vi "LV2 DVR Reference.vi"(0 "DVR Input":refnum<data-value>, 11 "Error in":errorcluster, 13 "Operation":T1) -> (4 "DVR Output":refnum<data-value>, 15 "Error out":errorcluster)   [LabVIEW 2020, in "DVR Access.lvlib"]
uses:
  DVR Access.lvlib
  Typedefs/LV2 Operations.ctl
  Typedefs/Data Cluster.ctl
  DVR Handson.lvlib
panel:
  # "LV2 DVR REFRENCE"
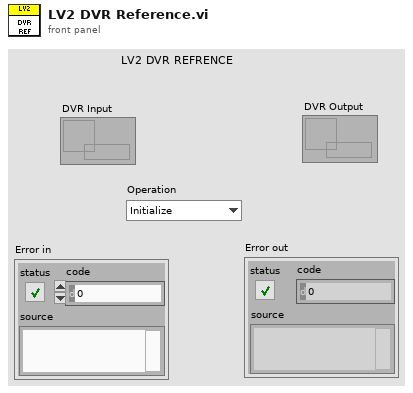
[diagram p1: front panel]
types:
  T1 = typedef "DVR Handson.lvlib/LV2 Operations.ctl" = enum16{"Initialize", "Read", "Write"}
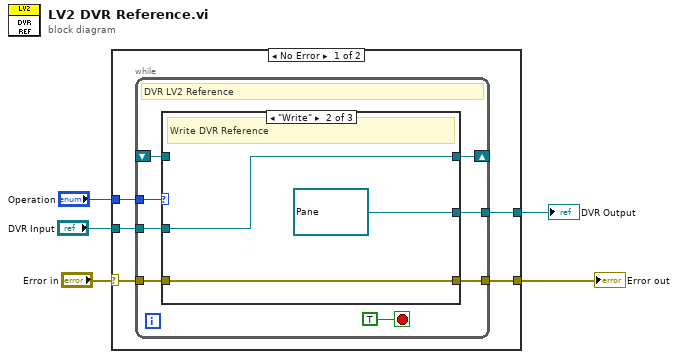
[diagram p0: block diagram]
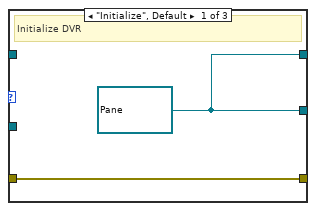
[diagram p2: hidden frame]
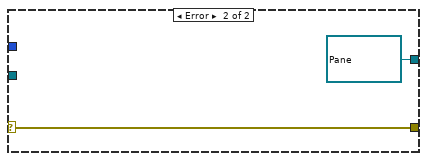
[diagram p4: hidden frame]
diagram:
  n1 = case shown="No Error" "Error in" {
    selector: "Error in" -> [w9 w27]
    tunnel: [w8 w27] -> w3
    tunnel: "Operation" -> [w10 _]
    tunnel: [w7 refnum<data-value> refnum ("DVR Input")] -> w1
    tunnel: "DVR Input" -> [w6 _]
    frame No Error {
      n2 = while {
        tunnel: w10 -> [w17]
        shift-right: [w13] -> _
        shift-left: _ -> [w11]
        tunnel: w9 -> [w16]
        tunnel: [w15] -> w8
        tunnel: [w14] -> w7
        tunnel: w6 -> [w12]
        stop <- TRUE stop-if-true
        # "DVR LV2 Reference"
        n3 = case shown="\"Write\"" w17 {
          tunnel: w16 -> [w20 w23 w25]
          tunnel: [w20 w23 w25] -> w15
          tunnel: [w19 refnum<data-value> refnum ("data value reference") w24] -> w14
          tunnel: [w19 w21 w24] -> w13
          tunnel: w12 -> [_ w21 _]
          tunnel: w11 -> [_ _ w24]
          frame "Initialize", Default {
            w19 = refnum<data-value> refnum ("data value reference")
            # "Initialize DVR"
          }
          frame "Write" {
            # "Write DVR Reference"
          }
          frame "Read" {
            # "Read DVR Reference"
          }
        }
      }
    }
    frame Error {
    }
  }
  "Error out" <- w3
  "DVR Output" <- w1
